vi "Get Target.vi"(6 "Axis":T1, 8 "error in (no error)":errorcluster, 11 "Instrument.VRM in":refnum<class "Instrument.OxfordVRM.lvclass">) -> (0 "error out":errorcluster, 1 "Target Field Rate (T/min)":dbl[](array[numeric]), 2 "Target Field (T)":dbl[](array[numeric]), 3 "Instrument.VRM out":refnum<class "Instrument.OxfordVRM.lvclass">)   [LabVIEW 2019, in "Instrument.OxfordVRM.lvclass"]
uses:
  Instrument.OxfordVRM.lvclass
  C:/Program Files (x86)/National Instruments/LabVIEW 2019/user.lib/LevyLab/Levylab Instruments/SMOs/Instrument/Instrument.lvclass
  Typedefs/VRM Magnet Axis--Enum.ctl
  Typedefs/Instrument.VRM.Commands-enum.ctl
  Typedefs/VRM Targets--Cluster.ctl
  <userlib>/LevyLab/Instrument Framework/SMOs/Instrument/Instrument.lvclass/Instrument.ctl
  fdec0842-03f0-4568-9df2-2b555409689a.vi
  fdec0842-03f0-4568-9df2-2b555409689a.vi/c32b0878-2925-4a8a-bedb-5aa7cbb350be.vi
  fdec0842-03f0-4568-9df2-2b555409689a.vi/c32b0878-2925-4a8a-bedb-5aa7cbb350be.vi/def422ff-bb17-4edd-abfe-315ab978a1c8.vi
  <userlib>/LevyLab/Instrument Framework/SMOs/Instrument/API/Send and Receive.vi
  fdec0842-03f0-4568-9df2-2b555409689a.vi/c32b0878-2925-4a8a-bedb-5aa7cbb350be.vi/def422ff-bb17-4edd-abfe-315ab978a1c8.vi/1f61b888-7954-489a-88a6-1f996c753a40.vi
  fdec0842-03f0-4568-9df2-2b555409689a.vi/c32b0878-2925-4a8a-bedb-5aa7cbb350be.vi/def422ff-bb17-4edd-abfe-315ab978a1c8.vi/26d63fa7-3c80-4ec1-8656-aae7aac92efd.vi
  <userlib>/LevyLab/Instrument Framework/SMOs/Instrument/API/Enum to String.vi
  <userlib>/LevyLab/Instrument Framework/SMOs/RemoteControl/API/Send and Receive.vi
  <vilib>/Utility/Data Type/Get Type Information.vi
  <vilib>/JDP Science/JSONtext/JSON text to Variant.vi
  <vilib>/JDP Science/JSONtext/LVClass Serializer/JSONtext LVClass Serializer.lvclass
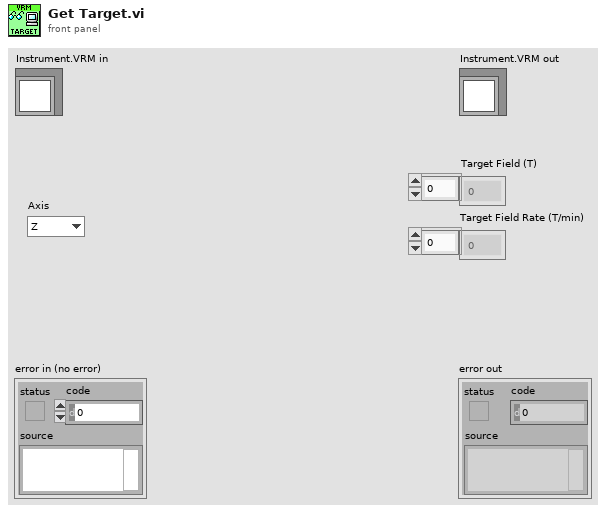
[diagram p1: front panel]
types:
  T1 = typedef "Instrument.OxfordVRM.lvclass/VRM Magnet Axis--Enum.ctl" = enum16{"Z", "X", "Y", "ALL"}
  T2 = typedef "Instrument.OxfordVRM.lvclass/VRM Targets--Cluster.ctl" = cluster{"Field (T)":dbl[], "Field Rate (T/min)":dbl[], "Axis":T1}
  T3 = typedef "Instrument.OxfordVRM.lvclass/Instrument.VRM.Commands-enum.ctl" = enum16{"setAction", "setTarget", "setMagnetField", "getStatus", "getTarget", "getMagnetField"}
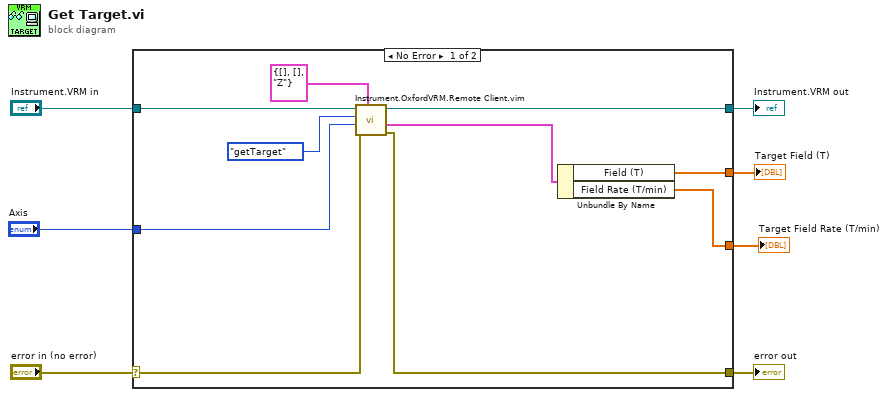
[diagram p0: block diagram]
diagram:
  n1 = case shown="No Error" "error in (no error)" {
    selector: "error in (no error)" -> [w16 w19]
    tunnel: [w15 w19] -> w6
    tunnel: [w11 w18] -> w4
    tunnel: "Instrument.VRM in" -> [w12 w18]
    tunnel: [w14 _] -> w3
    tunnel: [w13 _] -> w2
    tunnel: "Axis" -> [w9 _]
    frame No Error {
      n2 = call "Instrument.OxfordVRM.Remote Client.vim"("Data Out type"=T2 {"Field (T)"=[], "Field Rate (T/min)"=[], "Axis"=enum."Z"} ("Target"), "error in (no error)"=w16, "Data"=w9, "Commands"=Instrument.VRM.Commands-enum."getTarget", "Instrument.VRM in"=w12) -> ("error out"=w15:errorcluster, "Data out"=w10:T2, "Instrument.VRM out"=w11:refnum<class "Instrument.OxfordVRM.lvclass">)  [unwired: 4 in]
      n3 = Unbundle By Name(w10) -> ("Field (T)"=w14:dbl[], "Field Rate (T/min)"=w13:dbl[])
    }
    frame Error {
    }
  }
  "error out" <- w6
  "Instrument.VRM out" <- w4
  "Target Field (T)" <- w3
  "Target Field Rate (T/min)" <- w2
